vi "DataTransM2C.vi"(1 "MotorData":string) -> (0 "Computer Data":dbl[](array[numeric]))   [LabVIEW 2016]
doc: "This is a data transforming VI, from motor data to computer data."
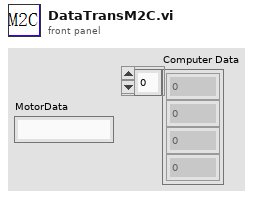
[diagram p1: front panel]
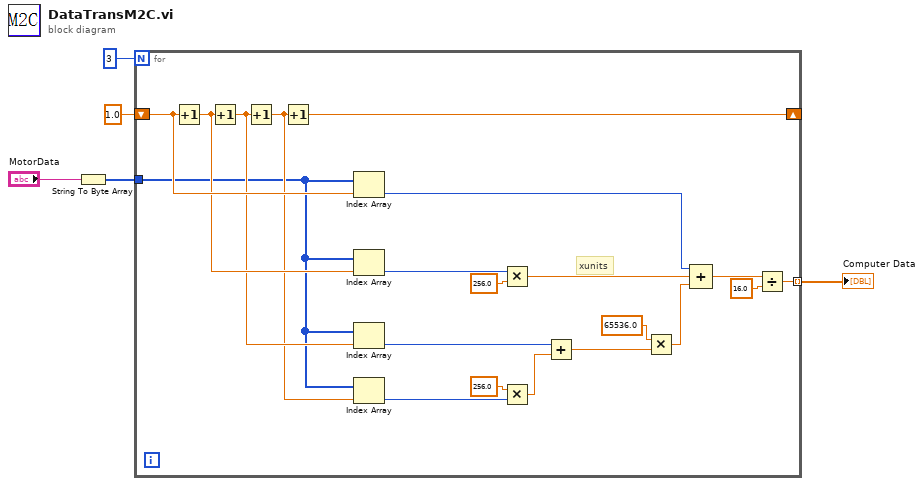
[diagram p0: block diagram]
diagram:
  n1 = String To Byte Array(string="MotorData") -> (unsigned byte array=w1:u8[])
  n2 = for {
    N: 3 -> [_]
    tunnel: [w16] -> w4 mode=indexing
    shift-right: [w15] -> _
    shift-left: 1.0 -> [w14]
    tunnel: w1 -> [w10]
    # "xunits"
    n3 = Increment(x=w14) -> (x+1=w13:dbl)
    n4 = Increment(x=w13) -> (x+1=w12:dbl)
    n5 = Increment(x=w12) -> (x+1=w11:dbl)
    n6 = Increment(x=w11) -> (x+1=w15:dbl)
    n7 = Index Array(array=w10, index=w14) -> (element=w9:u8)
    n8 = Index Array(array=w10, index=w13) -> (element=w8:u8)
    n9 = Index Array(array=w10, index=w12) -> (element=w7:u8)
    n10 = Index Array(array=w10, index=w11) -> (element=w6:u8)
    n11 = Multiply(x=w8, y=256.0) -> (x*y=w20:dbl)
    n12 = Multiply(x=256.0, y=w6) -> (x*y=w25:dbl)
    n13 = Add(x=w7, y=w25) -> (x+y=w24:dbl)
    n14 = Multiply(x=65536.0, y=w24) -> (x*y=w19:dbl)
    n15 = Compound Arithmetic op=ADD(w9, w20, w19) -> (w18:dbl)
    n16 = Divide(x=w18, y=16.0 ("x")) -> (x/y=w16:dbl)
  }
  "Computer Data" <- w4
